vi "Query Sequence Status.vi"(0 "VISA resource name":refnum<visa-resource-name>, 1 "Target Sync State (Adjusted)":i32(ring)=1 items=["Pending", "Adjusted"], 5 "Instance (1)":i32=1 format="%.0g", 7 "Timeout (1)":i32=1 format="%.0g", 9 "Target Main State (Run)":i32(ring)=1 items=["Off", "Run", "Ready"], 11 "error in (no error)":errorcluster) -> (4 "VISA resource name out":refnum<visa-resource-name>, 6 "Resources State":i32, 8 "Main State":i32, 10 "Sync State":i32, 15 "error out":errorcluster)   [LabVIEW 2015, in "Rohde&Schwarz CMXP GPRF.lvlib"]
doc: "Queries the main measurement state and the measurement substates.\n\nWithout query parameters, the states are returned immediately.\n\nWith query parameters, the states are returned when the <TargetMainState> and the <TargetSyncState> are reached or when the <Timeout> expires. \n\nAttribute(s):\nRSCMXPGPRF_ATTR_SEQUENCER_STATUS_ALL\n\nRemote-control command(s):\nSOURce:GPRF:GEN<i>:SEQuencer:STATe:ALL?"
uses:
  <instrlib>/Rohde&Schwarz CMXP GPRF/Rohde&Schwarz CMXP GPRF.lvlib
  <instrlib>/Rohde&Schwarz CMXP GPRF/Private/rsidr_core.llb/rsidr_core.lvlib
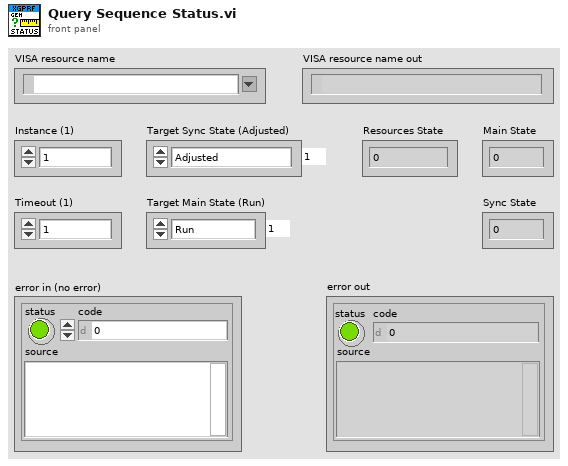
[diagram p1: front panel]
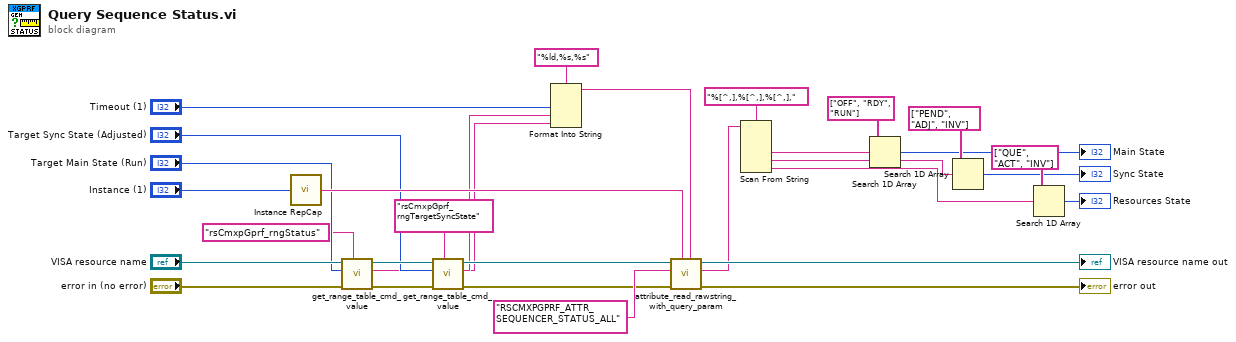
[diagram p0: block diagram]
diagram:
  n1 = call <instrlib>:"Instance RepCap.vi"("Instance in"="Instance (1)") -> ("Instance out"=w20:string)
  n2 = call <instrlib>:"get_range_table_cmd_value.vi"("Range Table ID in"="rsCmxpGprf_rngStatus", "error in"="error in (no error)", "Input Int32 value"="Target Main State (Run)", "VISA resource name"="VISA resource name") -> ("error out"=w17:errorcluster, "Cmd value out"=w7:string, "VISA resource name out"=w16:refnum<visa-resource-name>)  [unwired: 5 in]
  n3 = call <instrlib>:"get_range_table_cmd_value.vi"("Range Table ID in"="rsCmxpGprf_rngTargetSyncState", "error in"=w17, "Input Int32 value"="Target Sync State (Adjusted)", "VISA resource name"=w16) -> ("error out"=w15:errorcluster, "Cmd value out"=w6:string, "VISA resource name out"=w14:refnum<visa-resource-name>)  [unwired: 5 in]
  n4 = Format Into String(format string="%ld,%s,%s", "Timeout (1)", w7, w6) -> (resulting string=w1:string)  [unwired: 2 in, 1 out]
  n5 = call <instrlib>:"attribute_read_rawstring_with_query_param.vi"("Query Parameter (None)"=w1, "Repeated Capability (\"\")"=w20, "error in"=w15, "Attribute ID"="RSCMXPGPRF_ATTR_SEQUENCER_STATUS_ALL", "VISA resource name"=w14) -> ("error out"=→"error out":errorcluster, "RawString out"=w2:string, "VISA resource name out"=→"VISA resource name out":refnum<visa-resource-name>)  [unwired: 4 in]
  n6 = Scan From String(format string="%[^,],%[^,],%[^,],", input string=w2) -> (output 1=w30:string, output 2=w4:string, output 3=w3:string)  [unwired: 5 in, 3 out]
  n7 = Search 1D Array(1D array=string[] ["OFF", "RDY", "RUN"], element=w30) -> (index of element=→"Main State":i32)  [unwired: 1 in]
  n8 = Search 1D Array(1D array=string[] ["PEND", "ADJ", "INV"], element=w4) -> (index of element=→"Sync State":i32)  [unwired: 1 in]
  n9 = Search 1D Array(1D array=string[] ["QUE", "ACT", "INV"], element=w3) -> (index of element=→"Resources State":i32)  [unwired: 1 in]
